vi "rd_readData.vi"(6 "record start":u64, 7 "record index":u32, 8 "error in (no error)":errorcluster, 9 "length":u64, 11 "Excel refnum":T3) -> (0 "error out":errorcluster, 2 "real length":u64, 3 "data_AllTypeData":T1)   [LabVIEW 2020, in "NI_ExcelFile.lvlib"]
uses:
  <vilib>/express/express shared/NI_ExcelFile/NI_ExcelFile.lvlib
  <vilib>/express/express shared/NI_ExcelFile/Ctrls/ExcelRefnum.ctl
  <vilib>/express/express shared/NI_ExcelFile/Ctrls/MainData.ctl
  <vilib>/express/express shared/NI_ExcelFile/Ctrls/StreamMode.ctl
  <vilib>/express/express shared/NI_ExcelFile/Ctrls/TimeColumnMode.ctl
  <vilib>/express/express shared/NI_ExcelFile/Ctrls/FileAttribute.ctl
  <vilib>/express/express shared/NI_ExcelFile/Ctrls/Columns.ctl
  <vilib>/express/express shared/NI_ExcelFile/Ctrls/ColumnInfo.ctl
  <vilib>/express/express shared/NI_ExcelFile/Ctrls/DataType.ctl
  <vilib>/express/express shared/NI_ExcelFile/Ctrls/wd_recordInfo.ctl
  <vilib>/express/express shared/NI_ExcelFile/Ctrls/disk_TemplateFile.ctl
  <vilib>/express/express shared/NI_ExcelFile/Ctrls/meta_file.ctl
  <vilib>/express/express shared/NI_ExcelFile/Ctrls/meta_Block.ctl
  <vilib>/express/express shared/NI_ExcelFile/Ctrls/meta_BlockType.ctl
  <vilib>/express/express shared/NI_ExcelFile/Ctrls/data_AllTypeData.ctl
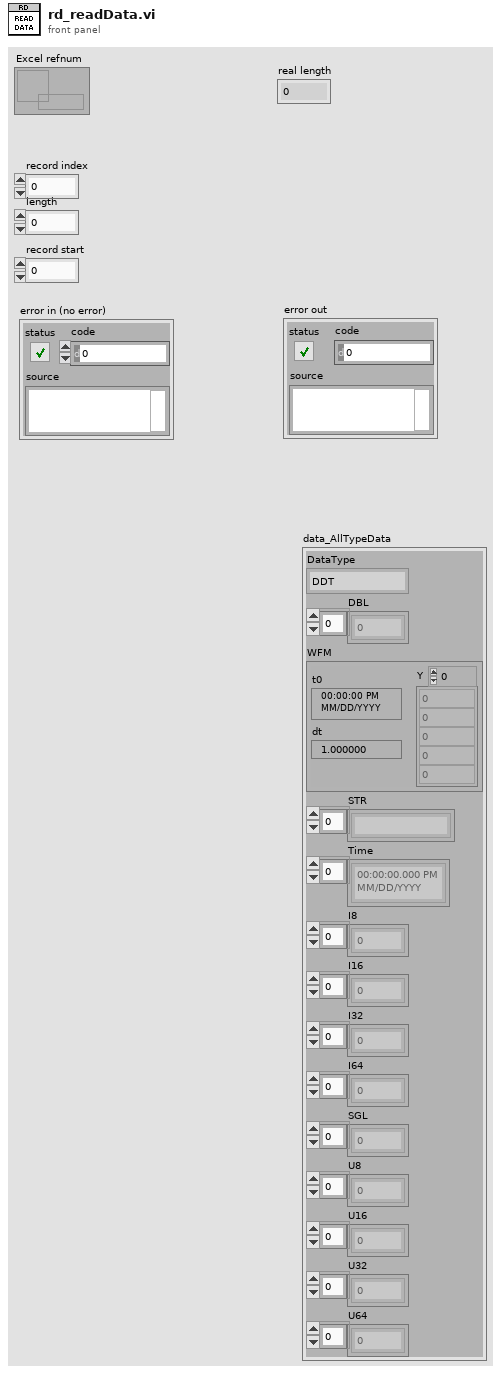
[diagram p1: front panel]
types:
  T1 = typedef "NI_ExcelFile.lvlib/data_AllTypeData.ctl" = cluster{"DataType":T2, "DBL":dbl[], "WFM":waveform(dbl), "STR":string[], "Time":timestamp[], "I8":i8[], "I16":i16[], "I32":i32[], "I64":i64[], "SGL":sgl[], "U8":u8[], "U16":u16[], "U32":u32[], "U64":u64[]}
  T2 = typedef "NI_ExcelFile.lvlib/DataType.ctl" = enum16{"DDT", "WFM", "Array of STR", "Array of DBL", "Array of I8", "Array of I16", "Array of I32", "Array of I64", "Array of SGL", "Array of U8", "Array of U16", "Array of U32", "Array of U64", "Array of Time"}
  T3 = typedef "NI_ExcelFile.lvlib/ExcelRefnum.ctl" = refnum<data-value>
  T4 = enum16{"column header", "column format", "column datatype", "column length"}
  T5 = typedef "NI_ExcelFile.lvlib/MainData.ctl" = cluster{"TargetFile":path, "StreamMode":T6, "Append?":bool, "ChunkSize":u64, "TimeColumnMode":T7, "TimestampFormat":string, "AbsoluteTime?":bool, "FileAttribute ":T8, "Column":T9, "FileRef":refnum<k1>, "MemoryRef":refnum<data-value>[], "RecordInfo":T11[], " ChannelPreviousInfo":u32[], "ChannelFirstRecord":u32[], "PredefinedFormattedValueLength":i64, "DiskTemplate":T12}
  T6 = typedef "NI_ExcelFile.lvlib/StreamMode.ctl" = enum16{"File", "Memory"}
  T7 = typedef "NI_ExcelFile.lvlib/TimeColumnMode.ctl" = enum16{"Empty", "OnePerCh", "One"}
  T8 = typedef "NI_ExcelFile.lvlib/FileAttribute.ctl" = cluster{"Creator":string, "Title":string, "SheetName":string}
  T9 = typedef "NI_ExcelFile.lvlib/Columns.ctl" = T10[]
  T10 = typedef "NI_ExcelFile.lvlib/ColumnInfo.ctl" = cluster{"Header":string, "Format":string, "DataType":T2, "Length":u64}
  T11 = typedef "NI_ExcelFile.lvlib/wd_recordInfo.ctl" = cluster{"ChannelIndex":u32, "StartIndex":u64, "Length":u64, "Previous":i32, "Next":i32}
  T12 = typedef "NI_ExcelFile.lvlib/disk_TemplateFile.ctl" = cluster{"XMLRef":refnum<file>[], "ZipPath":path, "MetaFile":T13, "TempFolder":path}
  T13 = typedef "NI_ExcelFile.lvlib/meta_file.ctl" = cluster{"Ref":refnum<file>, "NextRow":i32, "NextPosition":i64, "Block":T14[]}
  T14 = typedef "NI_ExcelFile.lvlib/meta_Block.ctl" = cluster{"Version":u16, "Type":T15, "Length":i32, "Data":string}
  T15 = typedef "NI_ExcelFile.lvlib/meta_BlockType.ctl" = enum16{"NITag", "File", "Column"}
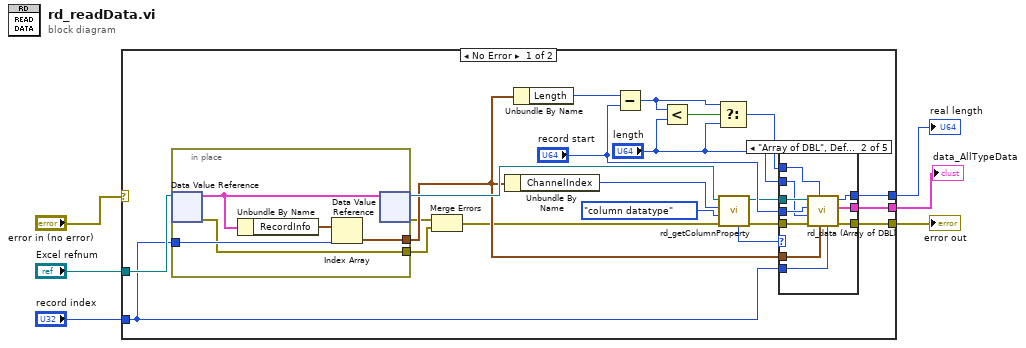
[diagram p0: block diagram]
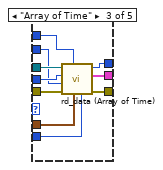
[diagram p3: hidden frame]
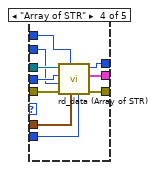
[diagram p4: hidden frame]
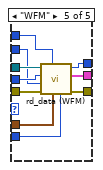
[diagram p5: hidden frame]
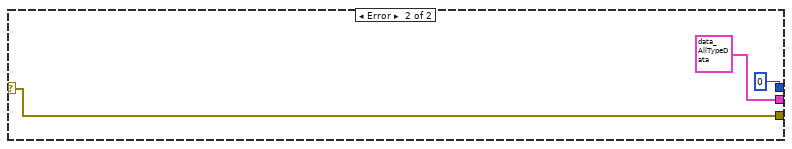
[diagram p6: hidden frame]
diagram:
  n1 = case shown="No Error" "error in (no error)" {
    selector: "error in (no error)" -> [_ w76]
    tunnel: [w26 w76] -> w6
    tunnel: [w25 u64 0 ("real length")] -> w5
    tunnel: "Excel refnum" -> [w14 _]
    tunnel: "record index" -> [w12 _]
    tunnel: [w7 T1 {"DataType"=enum."DDT", "DBL"=[], "WFM"={"t0"=timestamp(0 s since 1904-01-01), "dt"=1.0, "Y"=[]}, "STR"=[], "Time"=[], "I8"=[], "I16"=[], "I32"=[], "I64"=[], "SGL"=[], "U8"=[], "U16"=[], "U32"=[], "U64"=[]} ("fmt_AllTypeData")] -> w1
    frame No Error {
      n2 = in-place {
        in-place-border: w12 -> [w31]
        in-place-border: [w30] -> w11
        in-place-border: [w29] -> w8
        n3 = in-place-dvr #1(w14) -> (w28:T5, w29:errorcluster)
        n4 = Unbundle By Name(w28) -> ("RecordInfo"=w32:T11[])
        n5 = Index Array(array=w32, index=w31) -> (element=w30:T11)
        n6 = in-place-dvr #1(w28) -> (w13:T3, w9:errorcluster)
      }
      n7 = Merge Errors(w9, w8) -> (w10:errorcluster)
      n8 = Unbundle By Name(w11) -> ("ChannelIndex"=w19:u32)
      n9 = Unbundle By Name(w11) -> ("Length"=w21:u64)
      n10 = Subtract(x=w21, y="record start") -> (x-y=w20:u64)
      n11 = Less?(x=w20, y="length") -> (x < y?=w23:bool)
      n12 = Select(t=w20, s=w23, f="length") -> (s? t:f=w22:u64)
      n13 = call <vilib>:"rd_getColumnProperty.vi"("error in (no error)"=w10, "property"=T4."column datatype", "channel index"=w19, "Excel refnum"=w13) -> ("error out"=w15:errorcluster, "Excel refnum out"=w16:T3, "Column DataType"=w17:T2)  [unwired: 3 in, 2 out]
      n14 = case shown="\"Array of DBL\", Default" w17 {
        tunnel: "length" -> [_ w35 w45 w55 w65]
        tunnel: w22 -> [_ w34 w44 w54 w64]
        tunnel: w12 -> [_ w41 w51 w61 w71]
        tunnel: "record start" -> [_ w42 w52 w62 w72]
        tunnel: [_ w40 w50 w60 w70] -> w25
        tunnel: [w33 w38 w48 w58 w68] -> w26
        tunnel: [_ w39 w49 w59 w69] -> w7
        tunnel: w16 -> [_ w43 w53 w63 w73]
        tunnel: w11 -> [_ w37 w47 w57 w67]
        tunnel: w15 -> [w33 w36 w46 w56 w66]
        frame "DDT" {
        }
        frame "Array of DBL", Default {
          n15 = call <vilib>:"rd_data (Array of DBL).vi"("record index"=w41, "record info"=w37, "recordLenFromStart"=w34, "error in (no error)"=w36, "length"=w35, "record start"=w42, "ExcelRefnum"=w43) -> ("error out"=w38:errorcluster, "data_AllTypeData"=w39:T1, "real length"=w40:u64)  [unwired: 2 in]
        }
        frame "Array of Time" {
          n16 = call <vilib>:"rd_data (Array of Time).vi"("record index"=w51, "record info"=w47, "recordLenFromStart"=w44, "error in (no error)"=w46, "length"=w45, "record start"=w52, "ExcelRefnum"=w53) -> ("error out"=w48:errorcluster, "data_AllTypeData"=w49:T1, "real length"=w50:u64)  [unwired: 2 in]
        }
        frame "Array of STR" {
          n17 = call <vilib>:"rd_data (Array of STR).vi"("record index"=w61, "record info"=w57, "recordLenFromStart"=w54, "error in (no error)"=w56, "length"=w55, "record start"=w62, "ExcelRefnum"=w63) -> ("error out"=w58:errorcluster, "data_AllTypeData"=w59:T1, "real length"=w60:u64)  [unwired: 2 in]
        }
        frame "WFM" {
          n18 = call <vilib>:"rd_data (WFM).vi"("record index"=w71, "record info"=w67, "recordLenFromStart"=w64, "error in (no error)"=w66, "length"=w65, "record start"=w72, "ExcelRefnum"=w73) -> ("error out"=w68:errorcluster, "data_AllTypeData"=w69:T1, "real length"=w70:u64)  [unwired: 2 in]
        }
      }
    }
    frame Error {
    }
  }
  "error out" <- w6
  "real length" <- w5
  "data_AllTypeData" <- w1
